vi "告警码字段定义.vi"(7 "id":u16, 11 "告警代码":u16) -> (3 "报警":T1)   [LabVIEW 2016, in "斯坦道氨氮V2.lvlib"]
uses:
  Alarm interface/Alarm interface.lvlib
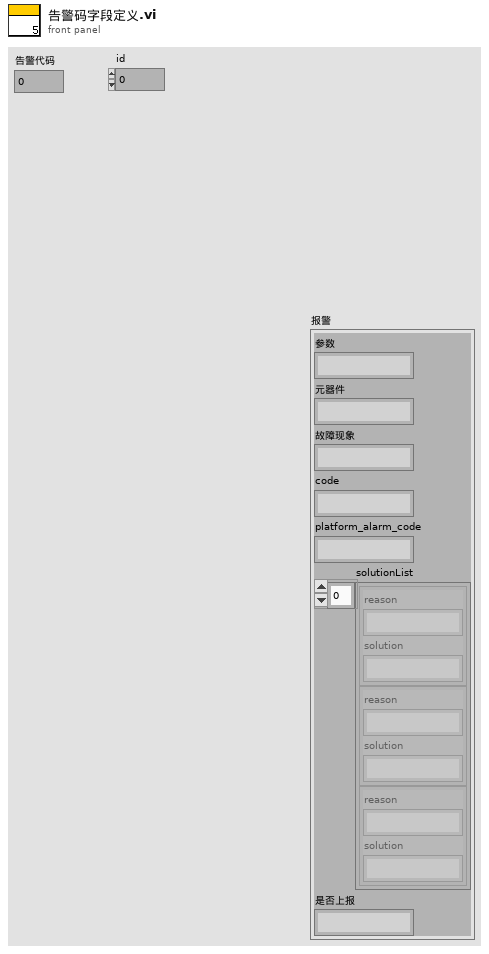
[diagram p1: front panel]
types:
  T1 = typedef "Alarm interface.lvlib/报警短信语音交互.ctl" = cluster{"参数":string, "元器件":string, "故障现象":string, "code":string, "platform_alarm_code":string, "solutionList":cluster{"reason":string, "solution":string}[], "是否上报":string}
  T2 = typedef "Alarm interface.lvlib/map in.ctl" = cluster{"name":string, "CN":string, "FirmwareVersion":string, "code":string}
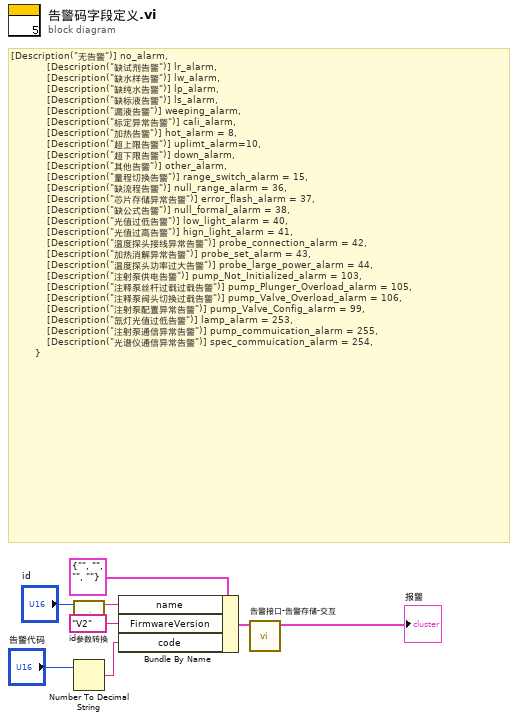
[diagram p0: block diagram]
diagram:
  # "[Description(\"无告警\")] no_alarm,\n            [Description(\"缺试剂告警\")] lr_alarm,\n            [Description(\"缺水样告警\")] lw_alarm,\n            [Description(\"缺纯水告警\")] lp_alarm,\n            [Description(\"缺标液告警\")] ls_alarm,\n            [Description(\"漏液告警\")] weeping_alarm,\n            [Description(\"标定异常告警\")] cali_alarm,\n            [Description(\"加热告警\")] hot_alarm = 8,\n            [Description(\"超上限告警\")] uplimt_alarm=10,\n            [Description(\"超下限告警\")] down_alarm,\n            [Description(\"其他告警\")] other_alarm,\n            [Description(\"量程切换告警\")] range_switch_alarm = 15,\n            [Description(\"缺流程告警\")] null_range_alarm = 36,\n            [Description(\"芯片存储异常告警\")] error_flash_alarm = 37,\n            [Description(\"缺公式告警\")] null_formal_alarm = 38,\n            [Description(\"光值过低告警\")] low_light_alarm = 40,\n            [Description(\"光值过高告警\")] hign_light_alarm = 41,\n            [Description(\"温度探头接线异常告警\")] probe_connection_alarm = 42,\n            [Description(\"加热消解异常告警\")] probe_set_alarm = 43,\n            [Description(\"温度探头功率过大告警\")] probe_large_power_alarm = 44,\n            [Description(\"注射泵供电告警\")] pump_Not_Initialized_alarm = 103,\n            [Description(\"注释泵丝杆过载过载告警\")] pump_Plunger_Overload_alarm = 105,\n            [Description(\"注释泵阀头切换过载告警\")] pump_Valve_Overload_alarm = 106,\n            [Description(\"注射泵配置异常告警\")] pump_Valve_Config_alarm = 99,\n            [Description(\"氙灯光值过低告警\")] lamp_alarm = 253,\n            [Description(\"注射泵通信异常告警\")] pump_commuication_alarm = 255,\n            [Description(\"光谱仪通信异常告警\")] spec_commuication_alarm = 254,\n        }"
  n1 = call "id参数转换.vi"("id"="id") -> ("table输出"=w7:string)  [unwired: 9 in, 1 out]
  n2 = Number To Decimal String(number="告警代码") -> (decimal integer string=w5:string)  [unwired: 1 in]
  n3 = Bundle By Name(cluster=T2 {"name"="", "CN"="", "FirmwareVersion"="", "code"=""} ("map in"), "name"=w7, "FirmwareVersion"="V2" ("equipVersion"), "code"=w5) -> (w1:T2)
  n4 = call "告警接口-告警存储-交互.vi"("map in"=w1) -> ("data"=→"报警":T1)  [unwired: 10 in]
